vi "Get Current Buffer.vi"() -> (2 "ZeroOffset":i32, 3 "Data":T1[](array[typedef]) {"Direction" items=["Tx", "Rx"]; "CANType" items=["CAN", "CANFD", "CANFD加速"]})   [LabVIEW 2018, in "CAN FD.lvlib"]
uses:
  CAN FD.lvlib
  Typedef/CAN Data.ctl
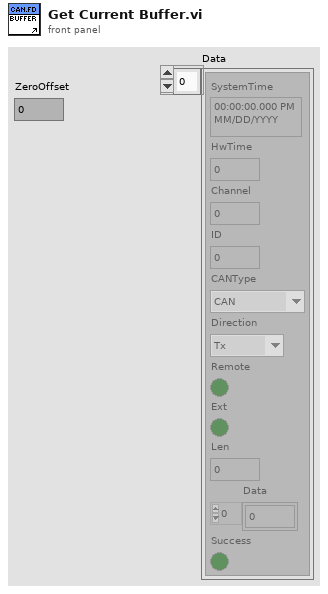
[diagram p1: front panel]
types:
  T1 = typedef "CAN FD.lvlib/CAN Data.ctl" = cluster{"SystemTime":timestamp, "HwTime":dbl, "Channel":u8, "ID":u32, "CANType":i16, "Direction":i16, "Remote":bool, "Ext":bool, "Len":u8, "Data":u8[], "Success":bool}
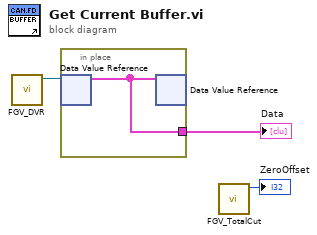
[diagram p0: block diagram]
diagram:
  n1 = call "FGV_DVR.vi"() -> ("DVR"=w3:refnum<data-value>)  [unwired: 10 in, 1 out]
  n2 = in-place {
    in-place-border: [w4] -> w2
    n3 = in-place-dvr #1(w3) -> (w4:T1[])  [unwired: 1 out]
    n4 = in-place-dvr #1(w4) -> ()  [unwired: 2 out]
  }
  "Data" <- w2
  n5 = call "FGV_TotalCut.vi"() -> ("Total cut"=→"ZeroOffset":i32)  [unwired: 10 in, 1 out]
